vi "Example Circular Buffer (Producer-Monitor).vi"() -> ()   [LabVIEW 2013]
uses:
  VariantBuffer/VariantBuffer.lvclass
panel:
  out "data":string[](array[string])
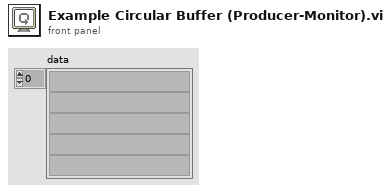
[diagram p1: front panel]
types:
  T1 = typedef "VariantBuffer.lvclass/buffer-event -- enum.ctl" = enum16{"element-added", "element-removed", "filled", "emptied", "resized", "default-changed", "destroyed"}
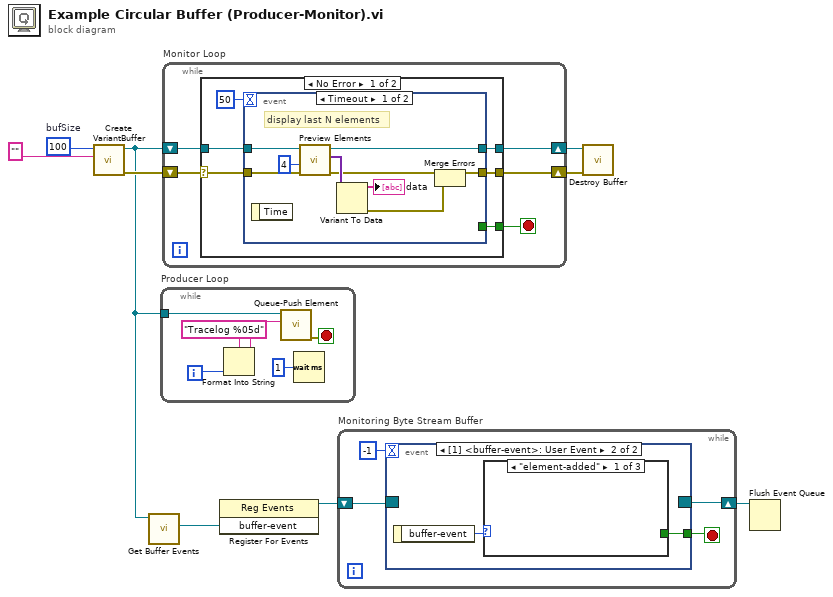
[diagram p0: block diagram]
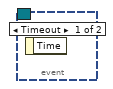
[diagram p2: hidden frame]
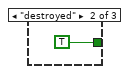
[diagram p3: hidden frame]
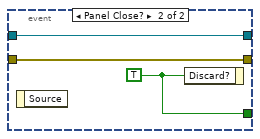
[diagram p5: hidden frame]
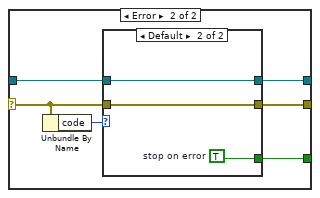
[diagram p6: hidden frame]
diagram:
  w9 = 100  # bufSize
  n1 = call "Create VariantBuffer.vi"("default"="", "bufSize"=w9) -> ("error out"=w6:errorcluster, "Buffer"=w1:refnum<data-value>)  [unwired: 8 in]
  n2 = call "Get Buffer Events.vi"("Buffer in"=w1) -> ("buffer-event"=w4:refnum<user-event>)  [unwired: 8 in, 2 out]
  n3 = while "Producer Loop" {
    tunnel: w1 -> [w12]
    i -> [w14]
    stop <- w10 stop-if-true
    n4 = Format Into String(format string="Tracelog %05d", w14) -> (resulting string=w11:string)  [unwired: 2 in, 1 out]
    n5 = call "Queue-Push Element.vi"("element"=w11, "Buffer in"=w12) -> ("error out"=w10:errorcluster)  [unwired: 6 in, 3 out]
    n6 = Wait (ms)(milliseconds to wait=u32 1) -> ()  [unwired: 1 out]
  }
  n7 = while "Monitor Loop" {
    shift-right: [w19] -> w7
    shift-left: w1 -> [w20]
    shift-right: [w18] -> w5
    shift-left: w6 -> [w16]
    stop <- w17 stop-if-true
    n8 = case shown="No Error" w16 {
      selector: w16 -> [w21 w40]
      tunnel: w20 -> [w25 w41]
      tunnel: [w24 w42] -> w19
      tunnel: [w23 w39] -> w18
      tunnel: [w22 w44] -> w17
      frame No Error {
        n9 = event shown="[0] Timeout" {
          selector: _ -> [_ _]
          dyn-events: _ -> [_ _]
          timeout: 50 -> [_ _]
          tunnel: w25 -> [w34 w38]
          tunnel: [w33 w38] -> w24
          tunnel: [_ w37] -> w22
          tunnel: w21 -> [w30 w36]
          tunnel: [w29 w36] -> w23
          event Timeout {
            # "display last N elements"
            n10 = event-data() -> ()  [unwired: 1 in, 1 out]
            n11 = call "Preview Elements.vi"("error in"=w30, "count (-1: all)"=4, "ByteBuffer in"=w34) -> ("error out"=w28:errorcluster, "elements"=w31:variant[], "ByteBuffer"=w33:refnum<data-value>)  [unwired: 6 in]
            n12 = Variant To Data(Variant=w31) -> (data=→"data":string[], error out=w27:errorcluster)  [unwired: 2 in]
            n13 = Merge Errors(w28, w27) -> (w29:errorcluster)
          }
          event Panel Close? {
            w37 = TRUE ("Discard?")
            n14 = event-data() -> ()  [unwired: 1 in, 1 out]
            n15 = event-data("Discard?"=w37) -> ()  [unwired: 1 in, 1 out]
          }
        }
      }
      frame Error {
        n16 = Unbundle By Name(w40) -> ("code"=w43:i32)
        n17 = case shown="Default" w43 {
          tunnel: [_ w48] -> w44
          tunnel: [w45 w47] -> w42
          tunnel: w41 -> [w45 w47]
          tunnel: w40 -> [_ w46]
          tunnel: [_ w46] -> w39
          frame 0 {
            # "Handle Error\n& Continue"
          }
          frame Default {
            w48 = TRUE  # stop on error
          }
        }
      }
    }
  }
  n18 = register-events(w4) -> (reference out=w3:refnum<event-registration>)  [unwired: 2 in, 1 out]
  n19 = while "Monitoring Byte Stream Buffer" {
    shift-right: [w50] -> w2
    shift-left: w3 -> [w51]
    stop <- w49 stop-if-true
    n20 = event shown="[1] <buffer-event>: User Event" {
      selector: w51 -> [_ _]
      dyn-events: [_ _] -> w50
      timeout: -1 -> [_ _]
      tunnel: [_ w53] -> w49
      event Timeout {
        n21 = event-data() -> ()  [unwired: 1 in, 1 out]
      }
      event User Event {
        n22 = event-data() -> ("buffer-event"=w54:T1)  [unwired: 1 in]
        n23 = case shown="\"element-added\"" w54 {
          tunnel: [_ TRUE _] -> w53
          frame "element-added" {
          }
          frame "destroyed" {
          }
          frame Default {
          }
        }
      }
    }
  }
  n24 = call "Destroy Buffer.vi"("error in"=w5, "Buffer"=w7) -> ()  [unwired: 8 in, 2 out]
  n25 = Flush Event Queue(0:w2) -> ()  [unwired: 5 in, 3 out]
